vi "SubSequenceUnpack.vi"(11 "input sequences":string[](array[string])) -> (3 "output sequences":string[](array[string]))   [LabVIEW 2019]
uses:
  <vilib>/Utility/file.llb/Read From Spreadsheet File (string).vi
panel:
  in  "stop":bool
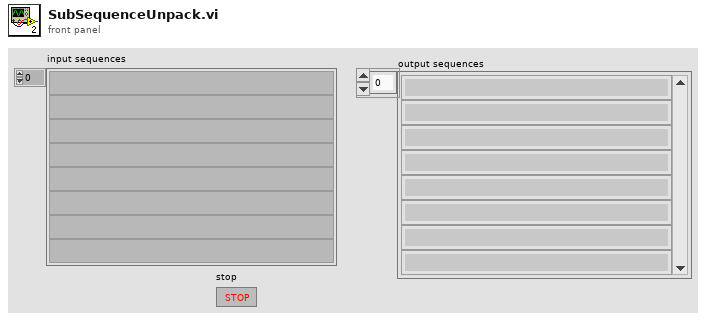
[diagram p1: front panel]
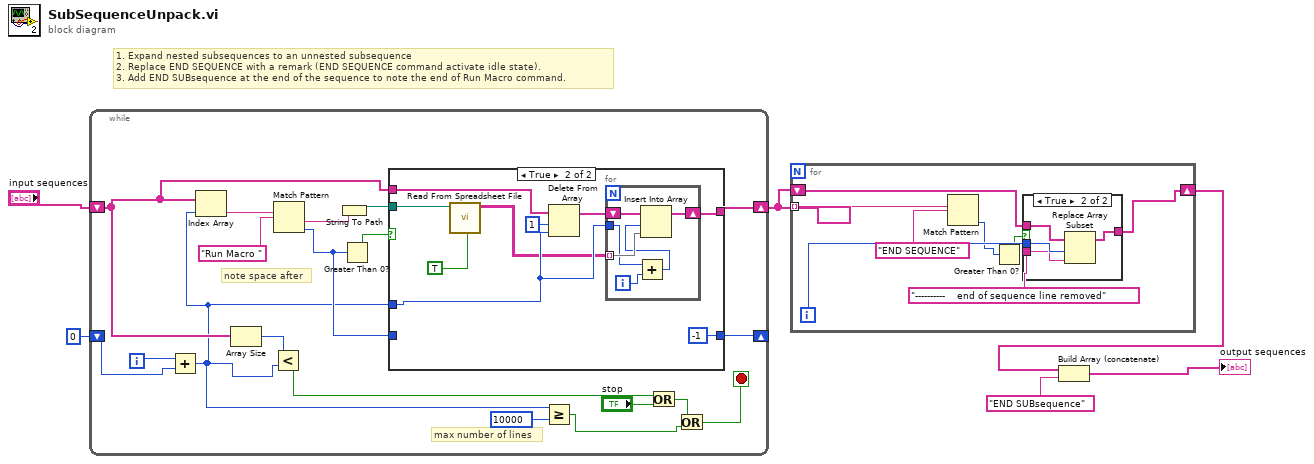
[diagram p0: block diagram]
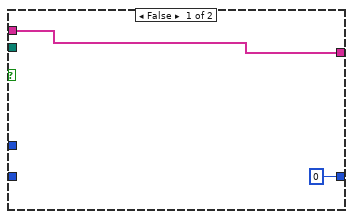
[diagram p3: hidden frame]
diagram:
  # "1. Expand nested subsequences to an unnested subsequence\n2. Replace END SEQUENCE with a remark (END SEQUENCE command activate idle state).\n3. Add END SUBsequence at the end of the sequence to note the end of Run Macro command."
  n1 = while {
    shift-right: [w20] -> w4
    shift-left: "input sequences" -> [w15]
    shift-right: [w18] -> _
    shift-left: 0 ("offset past match") -> [w16]
    i -> [w17]
    stop <- w7 stop-if-true
    # "max number of lines"
    # "note space after"
    n2 = Add(x=w17, y=w16) -> (x+y=w10:i32)
    n3 = Index Array(array=w15, index=w10) -> (element=w22:string)
    n4 = Array Size(array=w15) -> (size(s)=w14:i32)
    n5 = Less?(x=w14, y=w10) -> (x < y?=w13:bool)
    n6 = Match Pattern(string=w22, regular expression="Run Macro ") -> (after substring=w24:string, offset past match=w19:i32)  [unwired: 1 in, 2 out]
    n7 = String To Path(string=w24) -> (path=w23:path)
    n8 = Greater Than 0?(x=w19) -> (x > 0?=w21:bool)
    n9 = case shown="True" w21 {
      tunnel: w23 -> [_ w35]
      tunnel: w10 -> [_ w31]
      tunnel: w15 -> [w27 w34]
      tunnel: [w27 w29] -> w20
      tunnel: w19 -> [_ _]
      tunnel: [0 ("offset past match") -1 ("offset past match")] -> w18
      frame False {
      }
      frame True {
        n10 = call-poly <vilib>:"Read From Spreadsheet File.vi"("transpose (no:F)"=TRUE, "file path (dialog if empty)"=w35) -> ("all rows"=w30:string[][])  [unwired: 5 in, 4 out]
        n11 = Delete From Array(array=w34, length=1, index=w31) -> (array with subset deleted=w32:string[])  [unwired: 1 out]
        n12 = for {
          shift-right: [w38] -> w29
          shift-left: w32 -> [w42]
          tunnel: w31 -> [w39]
          tunnel: w30 -> [w41] mode=indexing
          i -> [w40]
          n13 = Add(x=w39, y=w40) -> (x+y=w37:i32)
          n14 = Insert Into Array(array=w42, index=w37, new element=w41) -> (w38:string[])
        }
      }
    }
    n15 = Greater Or Equal?(x=w10, y=10000) -> (x >= y?=w8:bool)
    n16 = Or(x=w13, y="stop") -> (x .or. y?=w11:bool)
    n17 = Or(x=w11, y=w8) -> (x .or. y?=w7:bool)
  }
  n18 = for {
    tunnel: w4 -> [w49] mode=indexing
    shift-right: [w45] -> w3
    shift-left: w4 -> [w46]
    i -> [w48]
    n19 = Match Pattern(string=w49, regular expression="END SEQUENCE") -> (offset past match=w44:i32)  [unwired: 1 in, 3 out]
    n20 = Greater Than 0?(x=w44) -> (x > 0?=w43:bool)
    n21 = case shown="True" w43 {
      tunnel: w48 -> [_ w55]
      tunnel: "----------    end of sequence line removed" ("result string") -> [_ w54]
      tunnel: w46 -> [w51 w53]
      tunnel: [w51 w52] -> w45
      frame False {
      }
      frame True {
        n22 = Replace Array Subset(array=w53, new element=w54, index=w55) -> (w52:string[])
      }
    }
  }
  n23 = Build Array (concatenate)(w3, "END SUBsequence" ("replace string (\"\")")) -> (→"output sequences":string[])
